vi "GE 5565PIORC.DMA.Scatter-Gather.vi"(10 "number of blocks (10)":i32=10, 11 "count per block (1000)":u32=1000) -> (0 "error out":errorcluster, 3 "pass?":bool)   [LabVIEW 2016]
uses:
  <vilib>/NI/GE Reflective Memory Driver/GE 5565PIORC.lvclass/GE 5565PIORC.ctl
  <vilib>/NI/GE Reflective Memory Driver/Methods/GE 5565PIORC.DMA.Block.Write (DBL).vi
  <vilib>/NI/GE Reflective Memory Driver/Methods/GE 5565PIORC.DMA.Create Transfer (Scatter-Gather).vi
  <vilib>/NI/GE Reflective Memory Driver/Methods/GE 5565PIORC.DMA.Block.Read (DBL).vi
  <vilib>/NI/GE Reflective Memory Driver/Properties/Registers/GE 5565PIORC.Registers.DMACSR0.Channel 0 Enable.Set.vi
  <vilib>/NI/GE Reflective Memory Driver/Properties/GE 5565PIORC.Read VISA MEMACC.vi
  <vilib>/NI/GE Reflective Memory Driver/Methods/GE 5565PIORC.DMA.Size.vi
  <vilib>/NI/GE Reflective Memory Driver/Methods/GE 5565PIORC.DMA.Configure.vi
  <vilib>/NI/GE Reflective Memory Driver/Methods/GE 5565PIORC.PXI Interrupts.Discard Events.vi
  <vilib>/NI/GE Reflective Memory Driver/Methods/GE 5565PIORC.DMA.Start.vi
  <vilib>/NI/GE Reflective Memory Driver/Methods/GE 5565PIORC.DMA.Interrupt.Wait for Done.vi
  <vilib>/NI/GE Reflective Memory Driver/Properties/Registers/GE 5565PIORC.Registers.Local Configuration.Read.vi
  <vilib>/NI/GE Reflective Memory Driver/Properties/Registers/GE 5565PIORC.Registers.Local Configuration.Read (U8).vi
  <vilib>/NI/GE Reflective Memory Driver/Properties/Registers/GE 5565PIORC.Registers.Local Configuration.Write.vi
  <vilib>/NI/GE Reflective Memory Driver/Properties/Registers/GE 5565PIORC.Registers.Local Configuration.Write (U8).vi
  <vilib>/NI/GE Reflective Memory Driver/Methods/GE 5565PIORC.Bit Manipulation.Set Bit.vi
  <vilib>/NI/GE Reflective Memory Driver/Methods/GE 5565PIORC.Bit Manipulation.Set Bit (U8).vi
  <vilib>/NI/GE Reflective Memory Driver/Properties/Registers/GE 5565PIORC.Registers.DMADPR0.Direction of Transfer.Set.vi
  <vilib>/NI/GE Reflective Memory Driver/Properties/Registers/GE 5565PIORC.Registers.DMASIZ0.DMA Transfer Size.Set.vi
  <vilib>/NI/GE Reflective Memory Driver/Properties/Registers/GE 5565PIORC.Registers.DMALADR0.Local Address Register.Set.vi
  <vilib>/NI/GE Reflective Memory Driver/Properties/Registers/GE 5565PIORC.Registers.DMAMODE0.Scatter-Gather Mode.Set.vi
  <vilib>/NI/GE Reflective Memory Driver/Properties/Registers/GE 5565PIORC.Registers.DMAPADR0.PCI Address Register.Set.vi
  <vilib>/NI/GE Reflective Memory Driver/Methods/GE 5565PIORC.DMA.Scatter-Gather.Link Block Descriptors.vi
  <vilib>/NI/GE Reflective Memory Driver/Methods/GE 5565PIORC.DMA.Scatter-Gather.Commit Linked Block Descriptors.vi
  <vilib>/NI/GE Reflective Memory Driver/Properties/Registers/GE 5565PIORC.Registers.DMADPR0.Channel 0 First Descriptor Address.Set.vi
  <vilib>/Utility/error.llb/Clear Errors.vi
  <vilib>/NI/GE Reflective Memory Driver/Properties/Registers/GE 5565PIORC.Registers.DMACSR0.Channel 0 Start.Set.vi
  <vilib>/NI/GE Reflective Memory Driver/Methods/GE 5565PIORC.PXI Interrupts.Wait for Event.vi
  <vilib>/NI/GE Reflective Memory Driver/Properties/Registers/GE 5565PIORC.Registers.DMACSR0.Channel 0 Clear Interrupt.Set.vi
  <vilib>/NI/GE Reflective Memory Driver/Methods/GE 5565PIORC.Registers.Read.vi
  <vilib>/NI/GE Reflective Memory Driver/Methods/GE 5565PIORC.Registers.Read (U8).vi
  <vilib>/NI/GE Reflective Memory Driver/Methods/GE 5565PIORC.Registers.Write.vi
  <vilib>/NI/GE Reflective Memory Driver/Methods/GE 5565PIORC.Registers.Write (U8).vi
  <vilib>/NI/GE Reflective Memory Driver/Properties/Registers/GE 5565PIORC.Registers.Local Configuration.Read (U32).vi
  <vilib>/NI/GE Reflective Memory Driver/Properties/Registers/GE 5565PIORC.Registers.Local Configuration.Write (U32).vi
  <vilib>/NI/GE Reflective Memory Driver/Methods/GE 5565PIORC.Bit Manipulation.Set Bit (U32).vi
  <vilib>/NI/GE Reflective Memory Driver/Methods/GE 5565PIORC.DMA.Scatter-Gather.Set Descriptor Params.vi
  <vilib>/NI/GE Reflective Memory Driver/Methods/GE 5565PIORC.Registers.Read (U32).vi
  <vilib>/NI/GE Reflective Memory Driver/Methods/GE 5565PIORC.Registers.Write (U32).vi
  <vilib>/NI/GE Reflective Memory Driver/Methods/GE 5565PIORC.Round Up to Nearest 8.vi
  <vilib>/NI/GE Reflective Memory Driver/Methods/GE 5565PIORC.Round Up to Nearest 16.vi
  <vilib>/NI/GE Reflective Memory Driver/GE 5565PIORC.lvclass
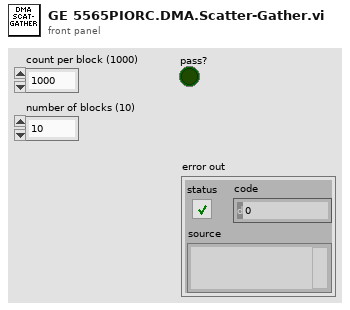
[diagram p1: front panel]
types:
  T1 = typedef "GE 5565PIORC.lvclass/GE 5565PIORC.Typedef.DMA Block Descriptor.ctl" = cluster{"descriptor ptr (VISA)":u32, "descriptor ptr (RFM)":u32, "descriptor size":u32, "descriptor params":T2}
  T2 = typedef "GE 5565PIORC.lvclass/GE 5565PIORC.Typedef.DMA Block Descriptor Params.ctl" = cluster{"data ptr (lower)":u32, "data ptr (upper)":u32, "data size":u32, "next descriptor ptr":u32}
  T3 = typedef "GE 5565PIORC.lvclass/GE 5565PIORC.Typedef.DMA Transfer Spec.ctl" = cluster{"RFM offset":u32, "Block Descriptors":T1[]}
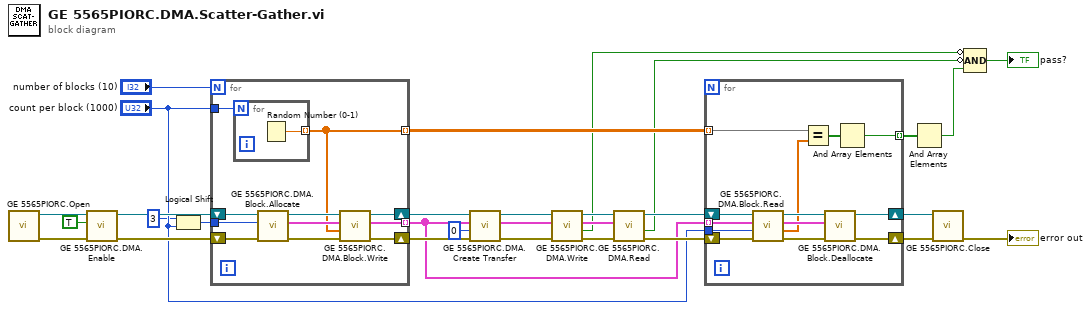
[diagram p0: block diagram]
diagram:
  n1 = call "GE 5565PIORC.Open.vi"() -> ("error out"=w25:errorcluster, "GE 5565PIORC"=w26:refnum<class "GE 5565PIORC.lvclass">)  [unwired: 10 in]
  n2 = call <vilib>:"GE 5565PIORC.DMA.Enable.vi"("error in (no error)"=w25, "enable (T)"=TRUE ("Enable DMA"), "GE 5565PIORC in"=w26) -> ("error out"=w27:errorcluster, "GE 5565PIORC out"=w28:refnum<class "GE 5565PIORC.lvclass">)  [unwired: 7 in]
  n3 = Logical Shift(y=i16 3, x="count per block (1000)") -> (x << y=w22:u32)
  n4 = for {
    N: "number of blocks (10)" -> [_]
    tunnel: [w34] -> w11 mode=indexing
    tunnel: "count per block (1000)" -> [w39]
    shift-right: [w33] -> w21
    shift-left: w28 -> [w41]
    shift-right: [w32] -> w20
    shift-left: w27 -> [w40]
    tunnel: w22 -> [w38]
    tunnel: [w31] -> w10 mode=indexing
    n5 = for {
      N: w39 -> [_]
      tunnel: [w42] -> w34 mode=indexing
      n6 = Random Number (0-1)() -> (number: 0 to 1=w42:dbl)
    }
    n7 = call <vilib>:"GE 5565PIORC.DMA.Block.Allocate.vi"("error in (no error)"=w40, "size in bytes"=w38, "GE 5565PIORC in"=w41) -> ("error out"=w36:errorcluster, "Block Descriptor"=w35:T1, "GE 5565PIORC out"=w37:refnum<class "GE 5565PIORC.lvclass">)  [unwired: 6 in]
    n8 = call-poly <vilib>:"GE 5565PIORC.DMA.Block.Write.vi"("error in (no error)"=w36, "data"=w34, "Block Descriptor in"=w35, "GE 5565PIORC in"=w37) -> ("error out"=w32:errorcluster, "Block Descriptor out"=w31:T1, "GE 5565PIORC out"=w33:refnum<class "GE 5565PIORC.lvclass">)  [unwired: 4 in, 1 out]
  }
  n9 = call-poly <vilib>:"GE 5565PIORC.DMA.Create Transfer.vi"("error in (no error)"=w20, "RFM offset"=u32 0, "Block Descriptors"=w10, "GE 5565PIORC in"=w21) -> ("error out"=w18:errorcluster, "DMA Transfer Spec"=w17:T3, "GE 5565PIORC out"=w19:refnum<class "GE 5565PIORC.lvclass">)  [unwired: 4 in, 1 out]
  n10 = call <vilib>:"GE 5565PIORC.DMA.Write.vi"("error in (no error)"=w18, "DMA Transfer Spec"=w17, "GE 5565PIORC in"=w19) -> ("error out"=w15:errorcluster, "timed out?"=w3:bool, "DMA Transfer Spec dup"=w14:T3, "GE 5565PIORC out"=w16:refnum<class "GE 5565PIORC.lvclass">)  [unwired: 5 in]
  n11 = call <vilib>:"GE 5565PIORC.DMA.Read.vi"("error in (no error)"=w15, "DMA Transfer Spec"=w14, "GE 5565PIORC in"=w16) -> ("error out"=w12:errorcluster, "timed out?"=w2:bool, "GE 5565PIORC out"=w13:refnum<class "GE 5565PIORC.lvclass">)  [unwired: 5 in, 1 out]
  n12 = for {
    shift-right: [w44] -> w6
    shift-left: w13 -> [w54]
    shift-right: [w43] -> w5
    shift-left: w12 -> [w53]
    tunnel: w11 -> [w51] mode=indexing
    tunnel: w10 -> [w55] mode=indexing
    tunnel: "count per block (1000)" -> [w52]
    tunnel: [w49] -> w7 mode=indexing
    n13 = call-poly <vilib>:"GE 5565PIORC.DMA.Block.Read.vi"("error in (no error)"=w53, "count"=w52, "Block Descriptor in"=w55, "GE 5565PIORC in"=w54) -> ("error out"=w47:errorcluster, "data out"=w45:dbl[], "Block Descriptor out"=w46:T1, "GE 5565PIORC out"=w48:refnum<class "GE 5565PIORC.lvclass">)  [unwired: 4 in]
    n14 = Equal?(x=w51, y=w45) -> (x = y?=w50:bool[])
    n15 = call <vilib>:"GE 5565PIORC.DMA.Block.Deallocate.vi"("error in (no error)"=w47, "Block Descriptor"=w46, "GE 5565PIORC in"=w48) -> ("error out"=w43:errorcluster, "GE 5565PIORC out"=w44:refnum<class "GE 5565PIORC.lvclass">)  [unwired: 7 in]
    n16 = And Array Elements(Boolean array=w50) -> (logical AND=w49:bool)
  }
  n17 = And Array Elements(Boolean array=w7) -> (logical AND=w4:bool)
  n18 = call "GE 5565PIORC.Close.vi"("error in (no error)"=w5, "GE 5565PIORC"=w6) -> ("error out"=→"error out":errorcluster)  [unwired: 9 in]
  n19 = Compound Arithmetic op=AND(invert w3, invert w2, w4) -> (→"pass?":bool)
